vi "Read Input Monitor Values.vi"(7 "Unit Address (1)":u8=1, 8 "error in (no error)":errorcluster, 10 "Selected Input Monitor (0: Input Monitor 1)":u8(ring) items=["Input monitor 1", "Input monitor 2"], 11 "VISA resource name":refnum<visa-resource-name>) -> (0 "error out":errorcluster, 1 "Minimum Recorded Input Since Last Reset":i32, 2 "Maximum Recorded Input Since Last Reset":i32, 3 "VISA resource name out":refnum<visa-resource-name>, 4 "Timer Threshold Value":i32)   [LabVIEW 2014, in "Eurotherm 35xx Series.lvlib"]
doc: "This VI returns Input Monitor Values."
uses:
  <instrlib>/Eurotherm 35xx Series/Eurotherm 35xx Series.lvlib
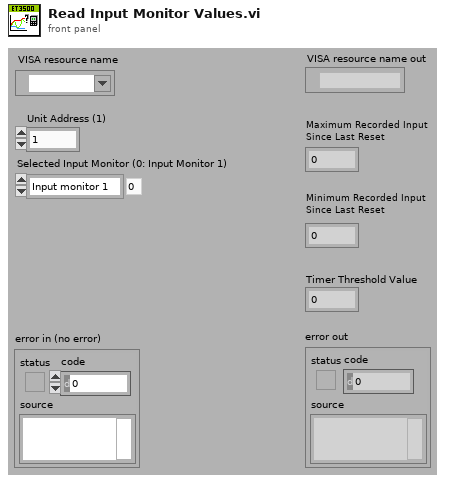
[diagram p1: front panel]
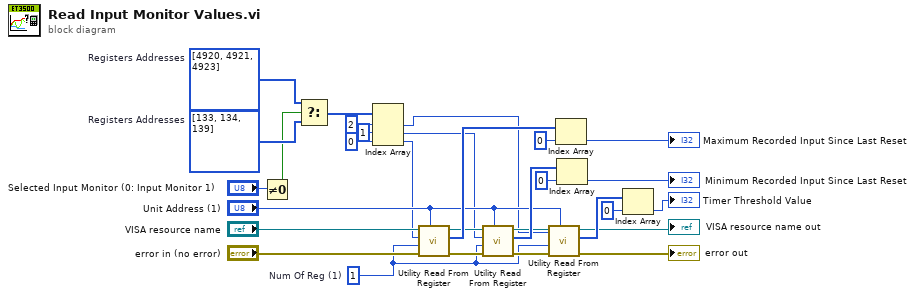
[diagram p0: block diagram]
diagram:
  w10 = u16[] [4920, 4921, 4923]  # Registers Addresses
  w11 = u16[] [133, 134, 139]  # Registers Addresses
  w18 = u16 1  # Num Of Reg (1)
  n1 = Not Equal To 0?(x="Selected Input Monitor (0: Input Monitor 1)") -> (x != 0?=w1:bool)
  n2 = Select(t=w10, s=w1, f=w11) -> (s? t:f=w9:u16[])
  n3 = Index Array(array=w9, index #1=2 ("index"), index #2=1 ("index"), index #3=0 ("index")) -> (element #1=w5:u16, element #2=w4:u16, element #3=w3:u16)
  n4 = call <instrlib>:"Utility Read From Register.vi"("Unit Address (1)"="Unit Address (1)", "error in (no error)"="error in (no error)", "Num Of Reg (1)"=w18, "Register Address (0)"=w3, "VISA resource name"="VISA resource name") -> ("error out"=w19:errorcluster, "Data"=w28:i16[], "VISA resource name out"=w22:refnum<visa-resource-name>)  [unwired: 4 in]
  n5 = call <instrlib>:"Utility Read From Register.vi"("Unit Address (1)"="Unit Address (1)", "error in (no error)"=w19, "Num Of Reg (1)"=w18, "Register Address (0)"=w4, "VISA resource name"=w22) -> ("error out"=w20:errorcluster, "Data"=w25:i16[], "VISA resource name out"=w21:refnum<visa-resource-name>)  [unwired: 4 in]
  n6 = call <instrlib>:"Utility Read From Register.vi"("Unit Address (1)"="Unit Address (1)", "error in (no error)"=w20, "Num Of Reg (1)"=w18, "Register Address (0)"=w5, "VISA resource name"=w21) -> ("error out"=→"error out":errorcluster, "Data"=w24:i16[], "VISA resource name out"=→"VISA resource name out":refnum<visa-resource-name>)  [unwired: 4 in]
  n7 = Index Array(array=w28, index=0) -> (element=→"Maximum Recorded Input Since Last Reset":i16)
  n8 = Index Array(array=w25, index=0) -> (element=→"Minimum Recorded Input Since Last Reset":i16)
  n9 = Index Array(array=w24, index=0) -> (element=→"Timer Threshold Value":i16)
